vi "Expo Scale Array.vi"(4 "Data":dbl[](array[numeric]), 5 "Params":dbl[](array[numeric])) -> (7 "Scaled Data":dbl[](array[numeric]))   [LabVIEW 2020, in "VolatusData.lvlib" / "Scaling.lvclass"]
uses:
  Scaling.lvclass
  Scaling.lvclass/Scaling.ctl
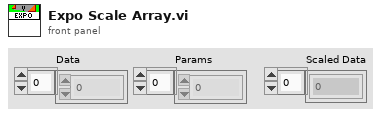
[diagram p1: front panel]
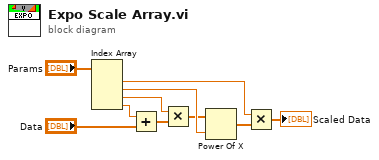
[diagram p0: block diagram]
diagram:
  n1 = Index Array(array="Params") -> (element #1=w2:dbl, element #2=w9:dbl, element #3=w5:dbl, element #4=w7:dbl)  [unwired: 4 in]
  n2 = Add(x=w7, y="Data") -> (x+y=w6:dbl[])
  n3 = Multiply(x=w5, y=w6) -> (x*y=w4:dbl[])
  n4 = Power Of X(1:w9, 2:w4) -> (0:w3:dbl[])
  n5 = Multiply(x=w2, y=w3) -> (x*y=→"Scaled Data":dbl[])
